vi "Back Initialize.vi"(1 "Back Right Close":u8=232, 2 "Back Right Open":u8=215, 3 "Back Left Close":u8=102, 4 "Back Left Open":u8=118) -> (0 "Back Grabber Total":T1)   [LabVIEW 2010, in "4150_RingItUp_State.lvrbt"]
uses:
  4150_RingItUp_State/4150_RingItUp_State.lvrbt
  Grabber Total.ctl
  <vilib>/NXT/Subs/MotorXNode.Servo Type.ctl
  grabber positions.ctl
  <vilib>/NXT/NXTIO Xnodes/AddressXNode/NXTIOAddress.xnode
  <vilib>/NXT/Subs/MotorXNode.1Servo.ctl
  <vilib>/NXT/Subs/LVHSConnector.ctl
  <vilib>/NXT/NXTIO Xnodes/NXTIOXNode/NXTIO.xnode
  <vilib>/NXT/NXTIO Xnodes/NXTIONodeSubVIs/TETRIX IO Move Servos.vi
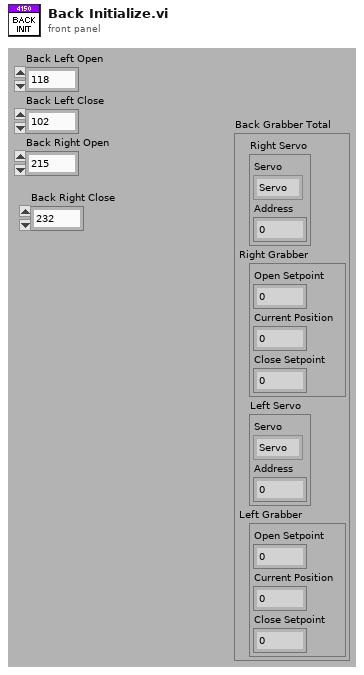
[diagram p1: front panel]
types:
  T1 = typedef "Grabber Total.ctl" = cluster{"Right Servo":cluster{"Servo":T2, "Address":i16}, "Right Grabber":T3, "Left Servo":cluster{"Servo":T2, "Address":i16}, "Left Grabber":T3}
  T2 = typedef "MotorXNode.Servo Type.ctl" = enum16{"Servo"}
  T3 = typedef "grabber positions.ctl" = cluster{"Open Setpoint":u8, "Current Position":u8, "Close Setpoint":u8}
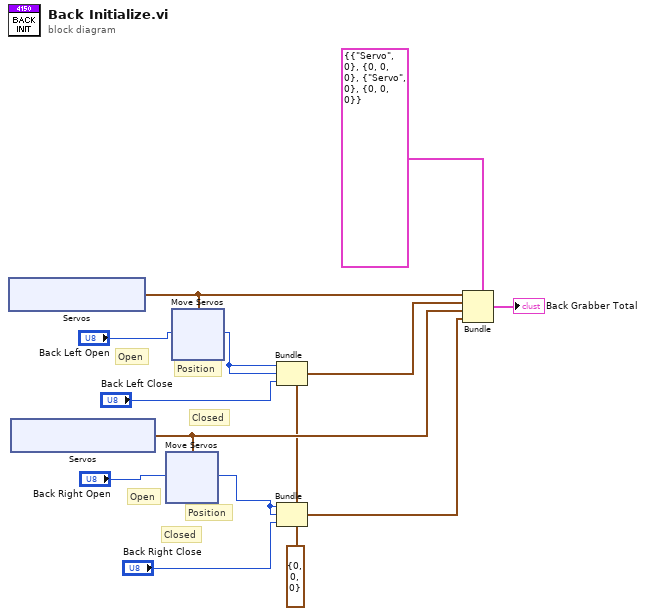
[diagram p0: block diagram]
diagram:
  w2 = T3 {"Open Setpoint"=0, "Current Position"=0, "Close Setpoint"=0} ("Left Grabber")
  # "Open"
  # "Closed"
  # "Position"
  # "Closed"
  # "Position"
  # "Open"
  n1 = xnode "Servos"() -> ("Servo"=w7:cluster{"Servo":T2, "Address":i16})
  n2 = xnode "Servos"() -> ("Servo"=w9:cluster{"Servo":T2, "Address":i16})
  n3 = xnode ("Move Servos")("Position 1"="Back Right Open", "Servos"=w9) -> ()  [unwired: 1 in, 1 out]
  n4 = xnode ("Move Servos")("Position 1"="Back Left Open", "Servos"=w7) -> ()  [unwired: 1 in, 1 out]
  n5 = Bundle(cluster=w2, "Open Setpoint"="Back Left Open", "Current Position"="Back Left Open", "Close Setpoint"="Back Left Close") -> (w8:T3)
  n6 = Bundle(cluster=w2, "Open Setpoint"="Back Right Open", "Current Position"="Back Right Open", "Close Setpoint"="Back Right Close") -> (w10:T3)
  n7 = Bundle(cluster=T1 {"Right Servo"={"Servo"=enum."Servo", "Address"=0}, "Right Grabber"={"Open Setpoint"=0, "Current Position"=0, "Close Setpoint"=0}, "Left Servo"={"Servo"=enum."Servo", "Address"=0}, "Left Grabber"={"Open Setpoint"=0, "Current Position"=0, "Close Setpoint"=0}}, "Right Servo"=w7, "Right Grabber"=w8, "Left Servo"=w9, "Left Grabber"=w10) -> (→"Back Grabber Total":T1)
